vi "Compose.vi"(8 "error in":errorcluster, 11 "Lv Proj Document Type:TAF Proj":refnum<class "TAF Proj.lvclass">) -> (0 "error out":errorcluster, 2 "Sections":refnum<class "Section.lvclass">[](array[class]), 3 "Lv Proj Document Type:TAF Proj":refnum<class "TAF Proj.lvclass">)   [LabVIEW 2021, in "TAF Proj Document Type.lvlib" / "TAF Proj.lvclass"]
uses:
  <vilib>/Wovalab/AntiDoc/Document Type/Add-ons/LabVIEW TAF Project/TAF Proj/TAF Proj.lvclass
  <vilib>/Wovalab/AntiDoc/Section/Section.lvclass
  <vilib>/Wovalab/AntiDoc/Document Type/Add-ons/LabVIEW TAF Project/TAF Proj/TAF Proj.lvclass/TAF Proj.ctl
  <vilib>/Wovalab/AntiDoc/Document Type/Add-ons/LabVIEW TAF Project/Project Parser/Target--cluster.ctl
  <vilib>/Wovalab/AntiDoc/Document Type/Add-ons/LabVIEW TAF Project/Project Parser/Blocs--cluster.ctl
  <vilib>/Wovalab/AntiDoc/Document Type/Add-ons/LabVIEW TAF Project/Dqmh Module/Dqmh Module.lvclass
  <vilib>/Wovalab/AntiDoc/Document Type/Add-ons/LabVIEW TAF Project/Class/Class.lvclass
  <vilib>/Wovalab/AntiDoc/Document Type/Add-ons/LabVIEW TAF Project/Lib/Lib.lvclass
  <vilib>/Wovalab/AntiDoc/Document Type/Add-ons/LabVIEW TAF Project/Custom Errors/Custom Errors.lvclass
  <vilib>/Wovalab/AntiDoc/Document Type/Add-ons/LabVIEW TAF Project/Classes Overview/Classes Overview.lvclass
  <vilib>/Wovalab/AntiDoc/Document Type/Add-ons/LabVIEW TAF Project/Dqmh Modules Overview/Dqmh Modules Overview.lvclass
  <vilib>/Wovalab/AntiDoc/Document Type/Add-ons/LabVIEW TAF Project/TAFConfiguration/TAFConfiguration.lvclass
  <vilib>/Wovalab/AntiDoc/Document Type/Add-ons/LabVIEW TAF Project/FrontPanelGUI/FrontPanelGUI.lvclass
  <vilib>/Wovalab/AsciiDoc for LabVIEW/Paragraph/Paragraph.lvclass
  C:/Program Files (x86)/National Instruments/LabVIEW 2021/vi.lib/Wovalab/AsciiDoc for LabVIEW/Adoc-Bloc/Bloc.lvclass
  <vilib>/Wovalab/AntiDoc/Bloc/Bloc.lvclass
  <vilib>/Wovalab/AntiDoc/Utilities/Utilities.lvlib
  <vilib>/Wovalab/AntiDoc/Document Type/Add-ons/LabVIEW TAF Project/Project Parser/Project Parser.lvlib
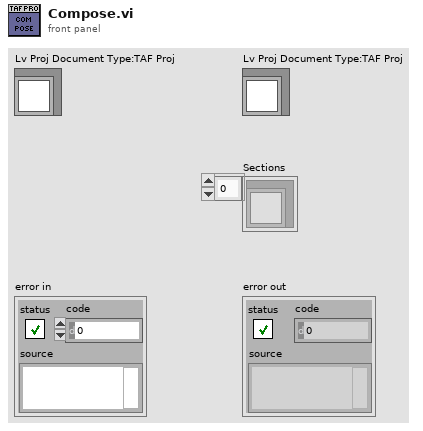
[diagram p1: front panel]
types:
  T1 = typedef "TAF Proj Document Type.lvlib/Project Parser.lvlib/Target--cluster.ctl" = cluster{"Name":string, "Blocs":T2}
  T2 = typedef "TAF Proj Document Type.lvlib/Project Parser.lvlib/Blocs--cluster.ctl" = cluster{"DQMH Modules":refnum<class "Dqmh Module.lvclass">[], "LVClasses":refnum<class "Class.lvclass">[], "Other Libraries":refnum<class "Lib.lvclass">[], "Custom Errors":refnum<class "Custom Errors.lvclass">, "Classes Overview":refnum<class "Classes Overview.lvclass">, "Dqmh Modules Overview":refnum<class "Dqmh Modules Overview.lvclass">, "TAFIFConfiguration":refnum<class "TAFConfiguration.lvclass">[], "FrontPanelGUIOut":refnum<class "FrontPanelGUI.lvclass">}
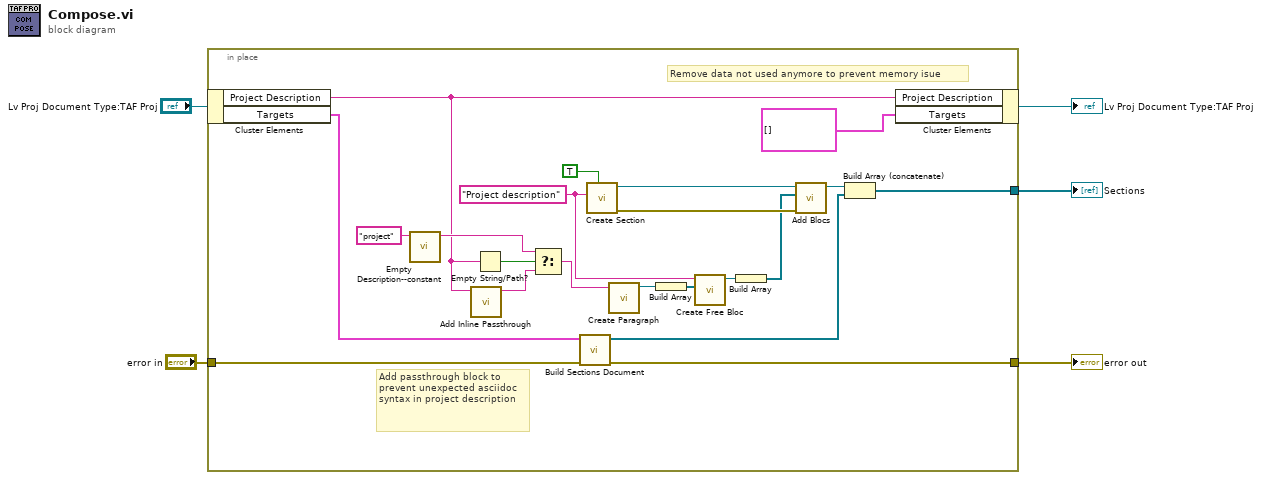
[diagram p0: block diagram]
diagram:
  n1 = in-place {
    in-place-border: [w26] -> w5
    in-place-border: "error in" -> [w25]
    in-place-border: [w14] -> w3
    w21 = "Project description" ("Name")
    # "Remove data not used anymore to prevent memory isue"
    # "Add passthrough block to prevent unexpected asciidoc syntax in project description"
    n2 = in-place-cluster #1("Lv Proj Document Type:TAF Proj") -> ("Project Description"=w6:string, "Targets"=w8:T1[])
    n3 = call <vilib>:"Empty Description--constant.vi"("Description Source"="project") -> ("Empty Description"=w10:string)  [unwired: 10 in]
    n4 = call <vilib>:"Add Inline Passthrough.vi"("String in"=w6) -> ("String out"=w9:string)  [unwired: 10 in]
    n5 = Empty String/Path?(string/path=w6) -> (empty?=w13:bool)
    n6 = Select(t=w10, s=w13, f=w9) -> (s? t:f=w12:string)
    n7 = call <vilib>:"Build Sections Document.vi"("error in"=w25, "Targets"=w8) -> ("error out"=w26:errorcluster, "Sections"=w15:refnum<class "Section.lvclass">[])  [unwired: 8 in]
    n8 = call <vilib>:"Create Section.vi"("No Title (F)"=TRUE, "Name"=w21) -> ("error out"=w24:errorcluster, "Section out"=w23:refnum<class "Section.lvclass">)  [unwired: 8 in]
    n9 = call <vilib>:"Create Paragraph.vi"("Content"=w12) -> ("Paragraph out"=w18:refnum<class "Paragraph.lvclass">)  [unwired: 9 in, 1 out]
    n10 = Build Array(w18) -> (w17:refnum<class "Paragraph.lvclass">[])
    n11 = call <vilib>:"Create Free Bloc.vi"("Content"=w17, "Name"=w21) -> ("Bloc out"=w20:refnum<class "Bloc.lvclass">)  [unwired: 8 in, 1 out]
    n12 = Build Array(w20) -> (w19:refnum<class "Bloc.lvclass">[])
    n13 = call <vilib>:"Add Blocs.vi"("error in (no error)"=w24, "Blocs"=w19, "Section in"=w23) -> ("Section out"=w16:refnum<class "Section.lvclass">)  [unwired: 7 in, 1 out]
    n14 = Build Array (concatenate)(w16, w15) -> (w14:refnum<class "Section.lvclass">[])
    n15 = in-place-cluster #1("Project Description"=w6, "Targets"=T1[] []) -> (→"Lv Proj Document Type:TAF Proj":refnum<class "TAF Proj.lvclass">)
  }
  "error out" <- w5
  "Sections" <- w3
